vi "get_lifterpara.vi"(8 "error in (no error)":errorcluster, 11 "configuration file path":path=path "E:/PHD/STF03/STF_Labview/Lifterconfig.ini") -> (0 "error out":errorcluster, 2 "Step possitions":dbl[](array[numeric]), 3 "ADC possitions":dbl[](array[numeric]))   [LabVIEW 2019]
uses:
  <vilib>/Utility/config.llb/Read Key (Double).vi
  <vilib>/Utility/config.llb/NI_LVConfig.lvlib
panel:
  out "element 3":dbl
  out "element 2":dbl
  out "element":dbl
  out "index of element":i32
  out "sorted array":dbl[](array[numeric])
  in  "new element/subarray":dbl
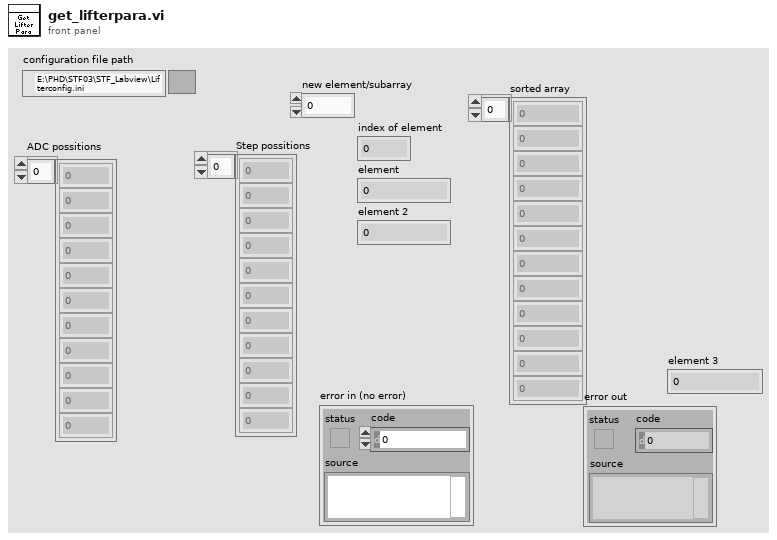
[diagram p1: front panel]
types:
  T1 = typedef "NI_LVConfig.lvlib/Config Data RefNum.ctl" = refnum<k1>
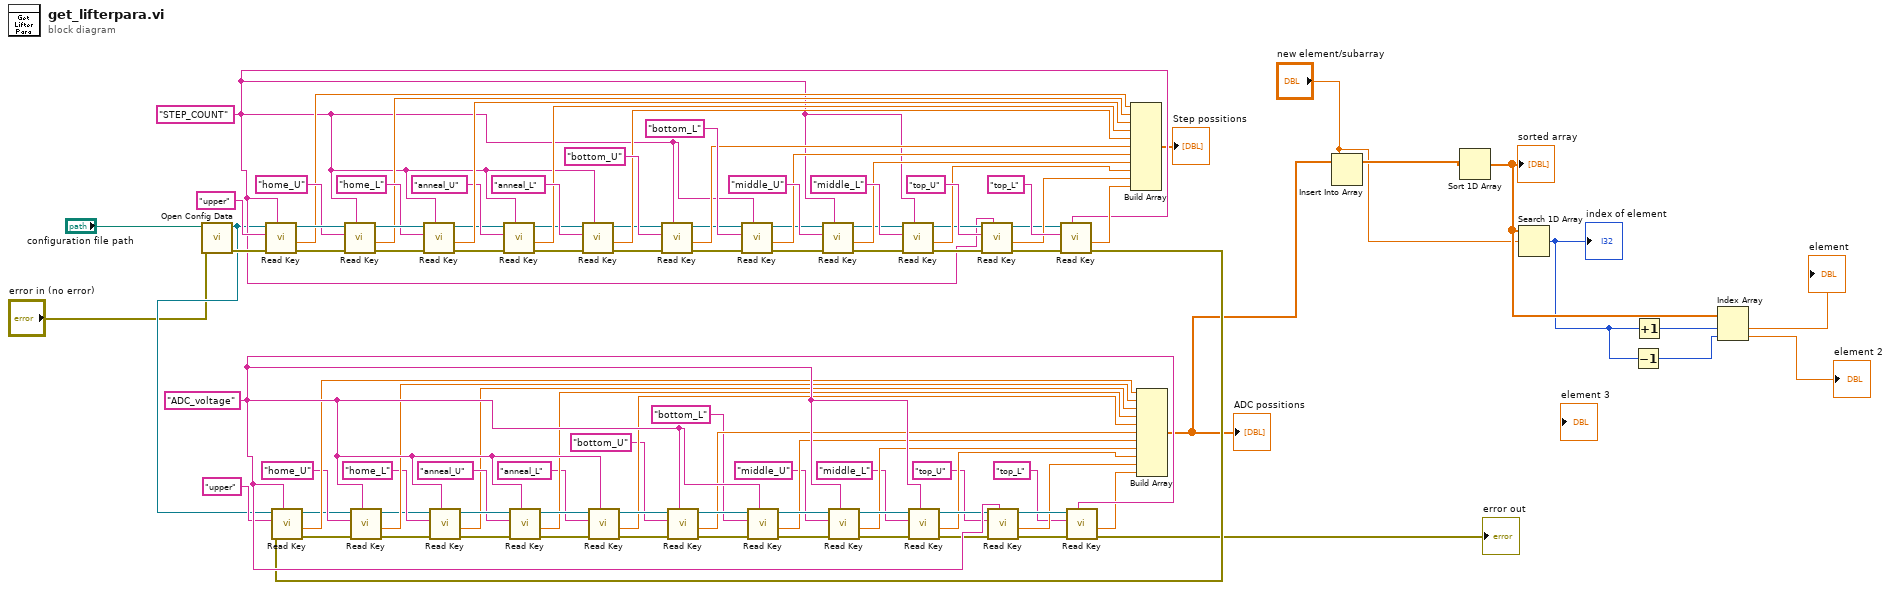
[diagram p0: block diagram]
diagram:
  w57 = "ADC_voltage" ("section")
  w58 = "STEP_COUNT" ("section")
  n1 = call <vilib>:"Open Config Data.vi"("error in (no error)"="error in (no error)", "configuration file path"="configuration file path") -> ("error out"=w100:errorcluster, "refnum"=w14:T1)  [unwired: 7 in, 1 out]
  n2 = call-poly <vilib>:"Read Key.vi"("section"=w58, "error in (no error)"=w100, "key"="upper", "refnum"=w14) -> ("error out"=w101:errorcluster, "value"=w93:dbl, "refnum out"=w102:T1)  [unwired: 4 in, 1 out]
  n3 = call-poly <vilib>:"Read Key.vi"("section"=w58, "error in (no error)"=w101, "key"="home_U", "refnum"=w102) -> ("error out"=w95:errorcluster, "value"=w92:dbl, "refnum out"=w96:T1)  [unwired: 4 in, 1 out]
  n4 = call-poly <vilib>:"Read Key.vi"("section"=w58, "error in (no error)"=w95, "key"="home_L", "refnum"=w96) -> ("error out"=w85:errorcluster, "value"=w91:dbl, "refnum out"=w66:T1)  [unwired: 4 in, 1 out]
  n5 = call-poly <vilib>:"Read Key.vi"("section"=w58, "error in (no error)"=w85, "key"="anneal_U", "refnum"=w66) -> ("error out"=w86:errorcluster, "value"=w74:dbl, "refnum out"=w65:T1)  [unwired: 4 in, 1 out]
  n6 = call-poly <vilib>:"Read Key.vi"("section"=w58, "error in (no error)"=w86, "key"="anneal_L", "refnum"=w65) -> ("error out"=w89:errorcluster, "value"=w73:dbl, "refnum out"=w64:T1)  [unwired: 4 in, 1 out]
  n7 = call-poly <vilib>:"Read Key.vi"("section"=w58, "error in (no error)"=w89, "key"="bottom_U", "refnum"=w64) -> ("error out"=w77:errorcluster, "value"=w72:dbl, "refnum out"=w63:T1)  [unwired: 4 in, 1 out]
  n8 = call-poly <vilib>:"Read Key.vi"("section"=w58, "error in (no error)"=w77, "key"="bottom_L", "refnum"=w63) -> ("error out"=w84:errorcluster, "value"=w71:dbl, "refnum out"=w62:T1)  [unwired: 4 in, 1 out]
  n9 = call-poly <vilib>:"Read Key.vi"("section"=w58, "error in (no error)"=w84, "key"="middle_U", "refnum"=w62) -> ("error out"=w83:errorcluster, "value"=w70:dbl, "refnum out"=w61:T1)  [unwired: 4 in, 1 out]
  n10 = call-poly <vilib>:"Read Key.vi"("section"=w58, "error in (no error)"=w83, "key"="middle_L", "refnum"=w61) -> ("error out"=w80:errorcluster, "value"=w69:dbl, "refnum out"=w60:T1)  [unwired: 4 in, 1 out]
  n11 = call-poly <vilib>:"Read Key.vi"("section"=w58, "error in (no error)"=w80, "key"="top_U", "refnum"=w60) -> ("error out"=w75:errorcluster, "value"=w68:dbl, "refnum out"=w59:T1)  [unwired: 4 in, 1 out]
  n12 = call-poly <vilib>:"Read Key.vi"("section"=w58, "error in (no error)"=w75, "key"="top_L", "refnum"=w59) -> ("error out"=w13:errorcluster, "value"=w67:dbl)  [unwired: 4 in, 2 out]
  n13 = call-poly <vilib>:"Read Key.vi"("section"=w57, "error in (no error)"=w13, "key"="upper", "refnum"=w14) -> ("error out"=w16:errorcluster, "value"=w22:dbl, "refnum out"=w15:T1)  [unwired: 4 in, 1 out]
  n14 = call-poly <vilib>:"Read Key.vi"("section"=w57, "error in (no error)"=w16, "key"="home_U", "refnum"=w15) -> ("error out"=w20:errorcluster, "value"=w23:dbl, "refnum out"=w19:T1)  [unwired: 4 in, 1 out]
  n15 = call-poly <vilib>:"Read Key.vi"("section"=w57, "error in (no error)"=w20, "key"="home_L", "refnum"=w19) -> ("error out"=w30:errorcluster, "value"=w24:dbl, "refnum out"=w49:T1)  [unwired: 4 in, 1 out]
  n16 = call-poly <vilib>:"Read Key.vi"("section"=w57, "error in (no error)"=w30, "key"="anneal_U", "refnum"=w49) -> ("error out"=w29:errorcluster, "value"=w41:dbl, "refnum out"=w50:T1)  [unwired: 4 in, 1 out]
  n17 = call-poly <vilib>:"Read Key.vi"("section"=w57, "error in (no error)"=w29, "key"="anneal_L", "refnum"=w50) -> ("error out"=w26:errorcluster, "value"=w42:dbl, "refnum out"=w51:T1)  [unwired: 4 in, 1 out]
  n18 = call-poly <vilib>:"Read Key.vi"("section"=w57, "error in (no error)"=w26, "key"="bottom_U", "refnum"=w51) -> ("error out"=w38:errorcluster, "value"=w43:dbl, "refnum out"=w52:T1)  [unwired: 4 in, 1 out]
  n19 = call-poly <vilib>:"Read Key.vi"("section"=w57, "error in (no error)"=w38, "key"="bottom_L", "refnum"=w52) -> ("error out"=w31:errorcluster, "value"=w44:dbl, "refnum out"=w53:T1)  [unwired: 4 in, 1 out]
  n20 = call-poly <vilib>:"Read Key.vi"("section"=w57, "error in (no error)"=w31, "key"="middle_U", "refnum"=w53) -> ("error out"=w32:errorcluster, "value"=w45:dbl, "refnum out"=w54:T1)  [unwired: 4 in, 1 out]
  n21 = call-poly <vilib>:"Read Key.vi"("section"=w57, "error in (no error)"=w32, "key"="middle_L", "refnum"=w54) -> ("error out"=w35:errorcluster, "value"=w46:dbl, "refnum out"=w55:T1)  [unwired: 4 in, 1 out]
  n22 = call-poly <vilib>:"Read Key.vi"("section"=w57, "error in (no error)"=w35, "key"="top_U", "refnum"=w55) -> ("error out"=w40:errorcluster, "value"=w47:dbl, "refnum out"=w56:T1)  [unwired: 4 in, 1 out]
  n23 = call-poly <vilib>:"Read Key.vi"("section"=w57, "error in (no error)"=w40, "key"="top_L", "refnum"=w56) -> ("error out"=→"error out":errorcluster, "value"=w48:dbl)  [unwired: 4 in, 2 out]
  n24 = Build Array(w93, w92, w91, w74, w73, w72, w71, w70, w69, w68, w67) -> (→"Step possitions":dbl[])
  n25 = Build Array(w22, w23, w24, w41, w42, w43, w44, w45, w46, w47, w48) -> (w3:dbl[])
  "ADC possitions" <- w3
  n26 = Insert Into Array(array=w3, new element="new element/subarray") -> (w12:dbl[])  [unwired: 1 in]
  n27 = Sort 1D Array(array=w12) -> (sorted array=w11:dbl[])
  "sorted array" <- w11
  n28 = Search 1D Array(1D array=w11, element="new element/subarray") -> (index of element=w8:i32)  [unwired: 1 in]
  "index of element" <- w8
  n29 = Decrement(x=w8) -> (x-1=w9:i32)
  n30 = Increment(x=w8) -> (x+1=w10:i32)
  n31 = Index Array(array=w11, index #1=w10, index #2=w9) -> (element #1=→"element":dbl, element #2=→"element 2":dbl)
